vi "MFC_Set - Revised.vi"(8 "error in":errorcluster, 10 "MFC info":T1={"MFC IDs"=["A", "B", "C", "D", "E"], "Setpoint"=[0.0, 0.0, 0.0, 0.0, 0.0], "Max Flow"=[1.0]}, 11 "VISA Session In":refnum<visa-resource-name>) -> (0 "error out":errorcluster, 2 "MFC_Data":string[](array[string]), 3 "VISA Sesssion Out":refnum<visa-resource-name>)   [LabVIEW 2019]
uses:
  <vilib>/Instr/_visa.llb/VISA Flush IO Buffer Mask.ctl
panel:
  out "Timing (ms)":u32
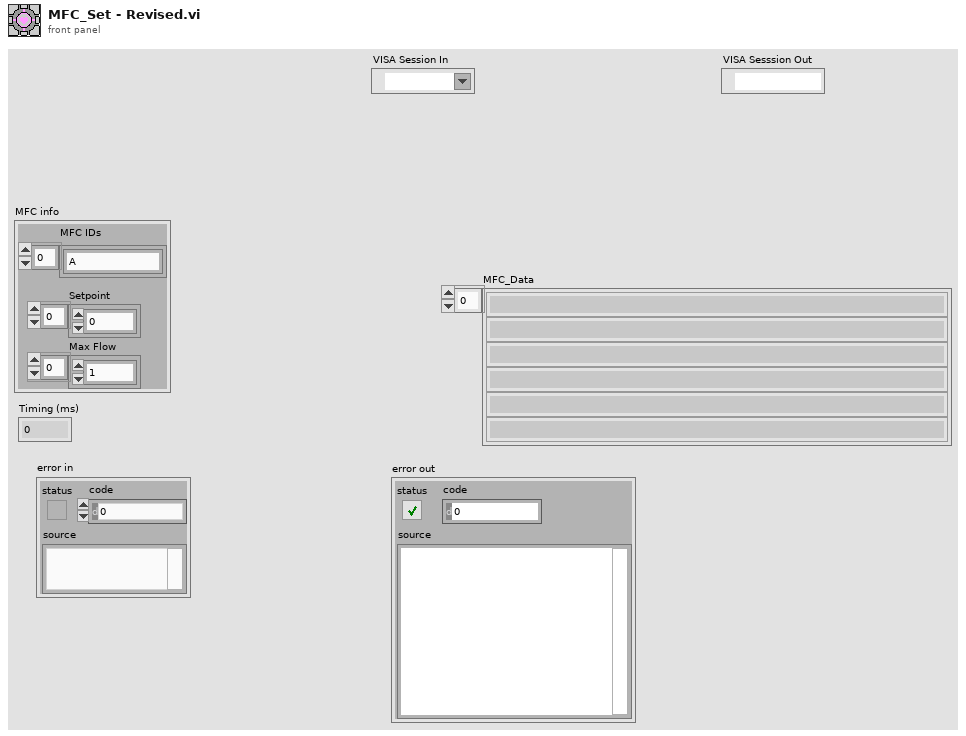
[diagram p1: front panel]
types:
  T1 = cluster{"MFC IDs":string[], "Setpoint":dbl[], "Max Flow":dbl[]}
  T2 = typedef "VISA Flush IO Buffer Mask.ctl" = u16
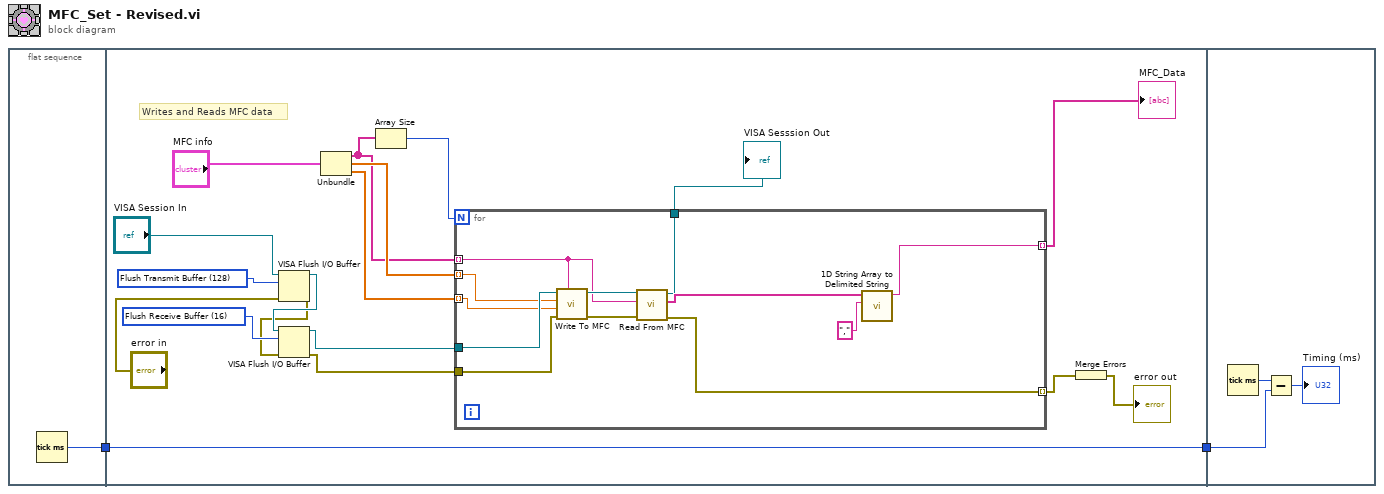
[diagram p0: block diagram]
diagram:
  n1 = flat-sequence {
    tunnel: [w3] -> w1
    tunnel: [w14] -> w2
    tunnel: w1 -> [w14]
    tunnel: w2 -> [w35]
    frame #0 {
      n2 = Tick Count (ms)() -> (millisecond timer value=w3:u32)
    }
    frame #1 {
      w10 = T2 16 items=["Flush Receive Buffer"=16, "Write Transmit Buffer to Device"=32, "Flush Receive Buffer (No I/O)"=64, "Flush Transmit Buffer"=128] ("Mask")
      w11 = T2 128 items=["Flush Receive Buffer"=16, "Write Transmit Buffer to Device"=32, "Flush Receive Buffer (No I/O)"=64, "Flush Transmit Buffer"=128] ("Mask")
      # "Writes and Reads MFC data"
      n3 = VISA Flush I/O Buffer(VISA resource name="VISA Session In", mask (16)=w11, error in (no error)="error in") -> (VISA resource name out=w8:refnum<visa-resource-name>, error out=w5:errorcluster)
      n4 = VISA Flush I/O Buffer(VISA resource name=w8, mask (16)=w10, error in (no error)=w5) -> (VISA resource name out=w7:refnum<visa-resource-name>, error out=w4:errorcluster)
      n5 = Unbundle("MFC info") -> ("MFC IDs"=w15:string[], "Setpoint"=w17:dbl[], "Max Flow"=w16:dbl[])
      n6 = Array Size(array=w15) -> (size(s)=w18:i32)
      n7 = for {
        N: w18 -> [_]
        tunnel: w7 -> [w32]
        tunnel: [w30] -> w20 mode=indexing
        tunnel: w17 -> [w28] mode=indexing
        tunnel: w16 -> [w27] mode=indexing
        tunnel: w15 -> [w29] mode=indexing
        tunnel: w4 -> [w26]
        tunnel: [w24] -> w13 mode=indexing
        tunnel: [w22] -> w12
        n8 = call "Write To MFC.vi"("Device ID (A)"=w29, "error in (no error)"=w26, "Device Range"=w27, "Set Point"=w28, "VISA Sesssion In"=w32) -> ("error out"=w31:errorcluster, "VISA Sesssion Out"=w33:refnum<visa-resource-name>)  [unwired: 3 in, 2 out]
        n9 = call "Read From MFC.vi"("error in (no error)"=w31, "Device ID"=w29, "VISA Sesssion In"=w33) -> ("error out"=w30:errorcluster, "Output"=w23:string[], "VISA Sesssion Out"=w22:refnum<visa-resource-name>)  [unwired: 6 in]
        n10 = call <vilib>:"1D String Array to Delimited String.vi"("delimiter"=",", "string array"=w23) -> ("delimited string"=w24:string)  [unwired: 9 in]
      }
      "MFC_Data" <- w13
      "VISA Sesssion Out" <- w12
      n11 = Merge Errors(w20) -> (→"error out":errorcluster)
    }
    frame #2 {
      n12 = Tick Count (ms)() -> (millisecond timer value=w36:u32)
      n13 = Subtract(x=w36, y=w35) -> (x-y=→"Timing (ms)":u32)
    }
  }
